vi "Error Handler.vi"(8 "error in":errorcluster, 11 "Alabama Power Remote in":refnum<class "Alabama Power Remote.lvclass">) -> (0 "error out":errorcluster, 3 "Alabama Power Remote out":refnum<class "Alabama Power Remote.lvclass">)   [LabVIEW 2018, in "Alabama Power Remote Actor.lvlib" / "Alabama Power Remote.lvclass"]
uses:
  Alabama Power Remote.lvclass
  <vilib>/Utility/error.llb/DialogType.ctl
  Utilities/Status Messaging.llb/Status Messaging.lvlib
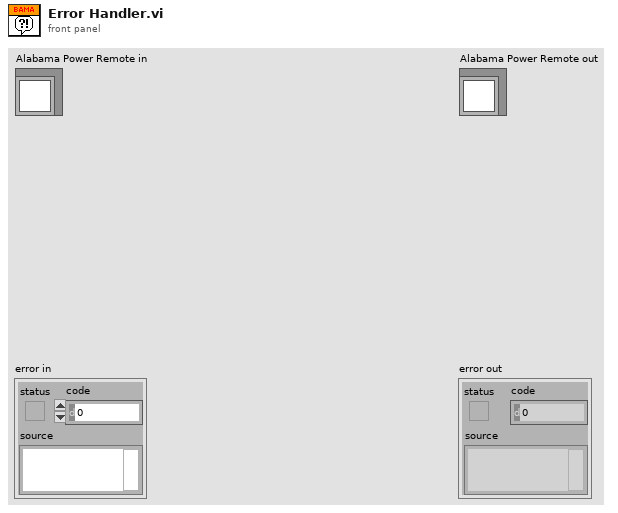
[diagram p1: front panel]
types:
  T1 = typedef "DialogType.ctl" = u16
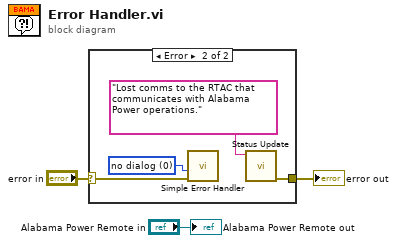
[diagram p0: block diagram]
diagram:
  n1 = case shown="Error" "error in" {
    selector: "error in" -> [w4 w8]
    tunnel: [w4 w6] -> w2
    frame No Error {
    }
    frame Error {
      w7 = T1 0 items=["no dialog", "OK message", "continue or stop message", "OK message + warnings", "continue/stop + warnings"] ("type of dialog (OK msg:1)")
      n2 = call <vilib>:"Simple Error Handler.vi"("type of dialog (OK msg:1)"=w7, "error in (no error)"=w8) -> ()  [unwired: 3 in, 5 out]
      n3 = call "Status Update.vi"("Status Update"="Lost comms to the RTAC that communicates with Alabama Power operations.") -> ("error out"=w6:errorcluster)  [unwired: 9 in, 1 out]
    }
  }
  "error out" <- w2
  "Alabama Power Remote out" <- "Alabama Power Remote in"
